vi "FTW-TestStep-Template-Core_Step.vi"(0 "FTW Actor Instance Configuration":string="{\n  \"Identity\": \"ActorName\",\n  \"InboxAddress\": \"inproc://*\",\n  \"LoggerAddress\": \"\",\n  \"My Data\": false,\n  \"Publisher URI\": \"inproc://*\",\n  \"Subscriber URIs\": \"\",\n  \"Refresh Period\": 2\n}", 11 "ErrorIn":errorcluster) -> (15 "Error":errorcluster)   [LabVIEW 2018, in "FTW-TestStep-Template-Core.lvclass"]
uses:
  FTW-TestStep-Template-Core.lvclass
  FTW-TestStep-Template-Core.lvclass/FTW-TestStep-Template-Core.ctl
  source/actor/Instance/FTW-ActorInstance.lvclass/FTW-ActorInstance.ctl
  5377bbb3-02f5-4951-b373-df4eba9c7bf2.vi
  5377bbb3-02f5-4951-b373-df4eba9c7bf2.vi/26df914e-262b-454c-b8ca-6c85922b0070.vi
  C:/Jobs/Featherweight/featherweight-2018/source/actor/Instance/FTW-ActorInstance.lvclass
  source/container/FTW-Container-FromVariant.vi
  source/container/FTW-Container-New-FromContainer.vi
  source/JSON/FTW-JSON-SerializeAndDestroy.vi
  source/actor/JobSequencer/FTW-SEQ-Current.vi
  source/actor/Message/Base/FTW-Message.lvclass
  source/actor/Connector/FTW-ActorConnector.lvclass
  source/actor/Instance/FTW-ActorInstance.lvclass
  source/actor/Message/Request/FTW-Message-IncomingRequest.lvclass
  source/actor/Publisher/FTW-Publisher.lvclass
  source/actor/Subscriber/FTW-Subscriber.lvclass
panel:
  # "#TODO\nhide controls for a GUI"
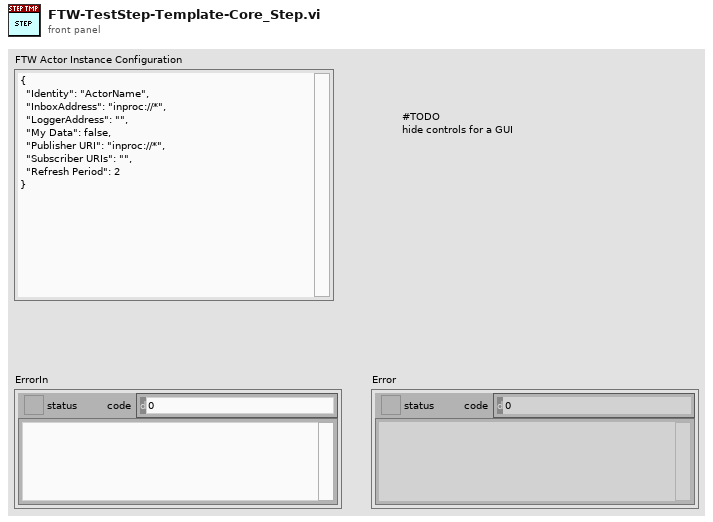
[diagram p1: front panel]
types:
  T1 = cluster{"Incoming Requests":refnum<event-registration>, "Local Messages":refnum<event-registration>, "Subscriber Registration":refnum<event-registration>}
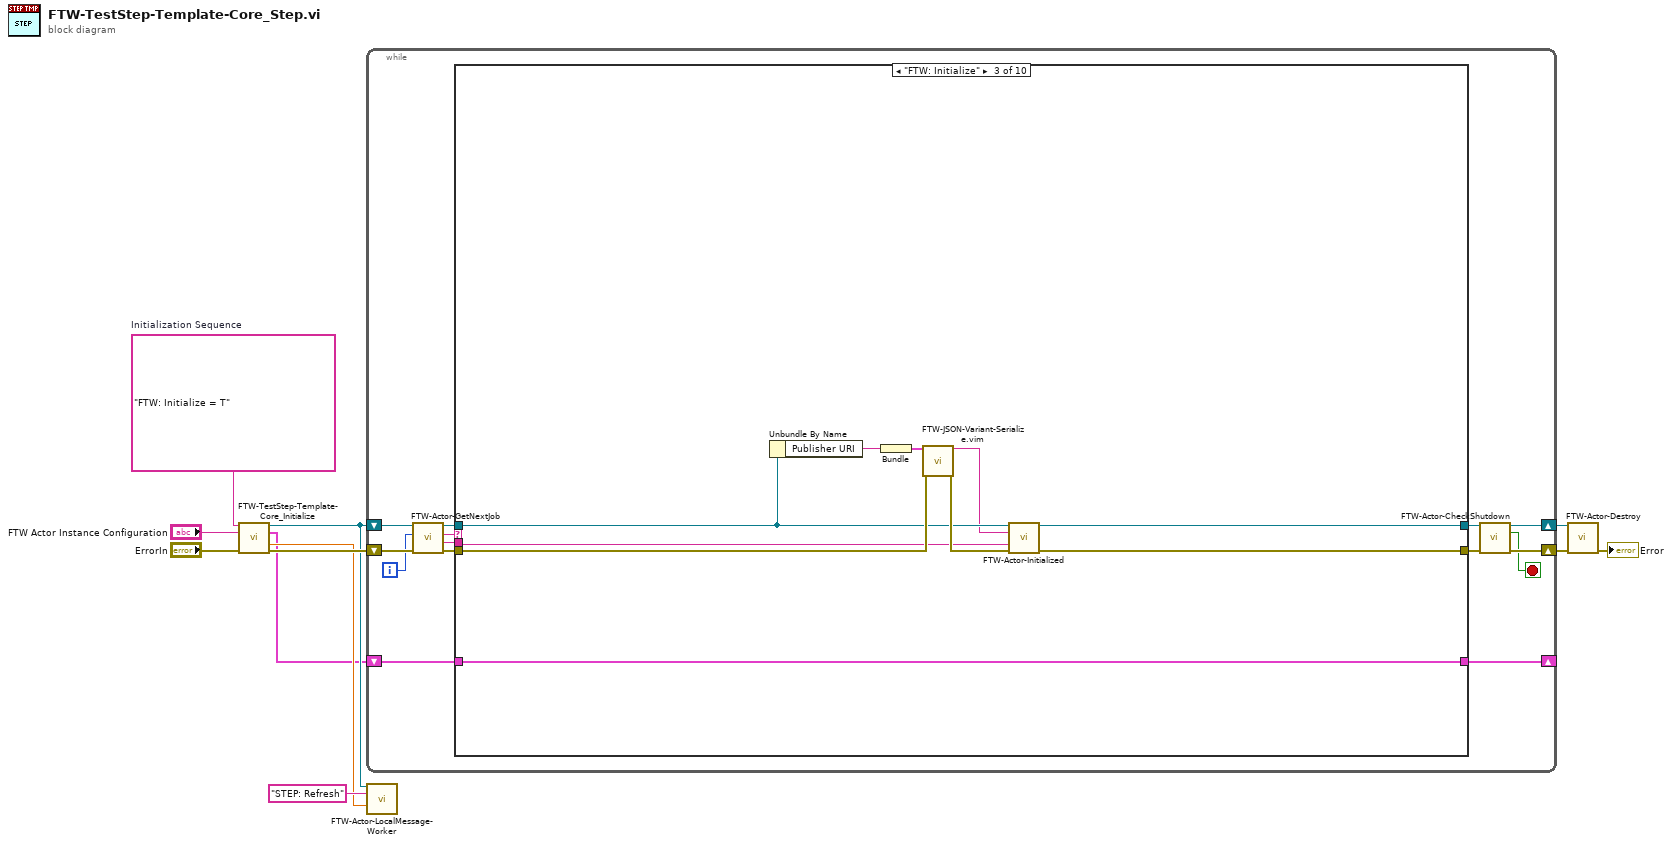
[diagram p0: block diagram]
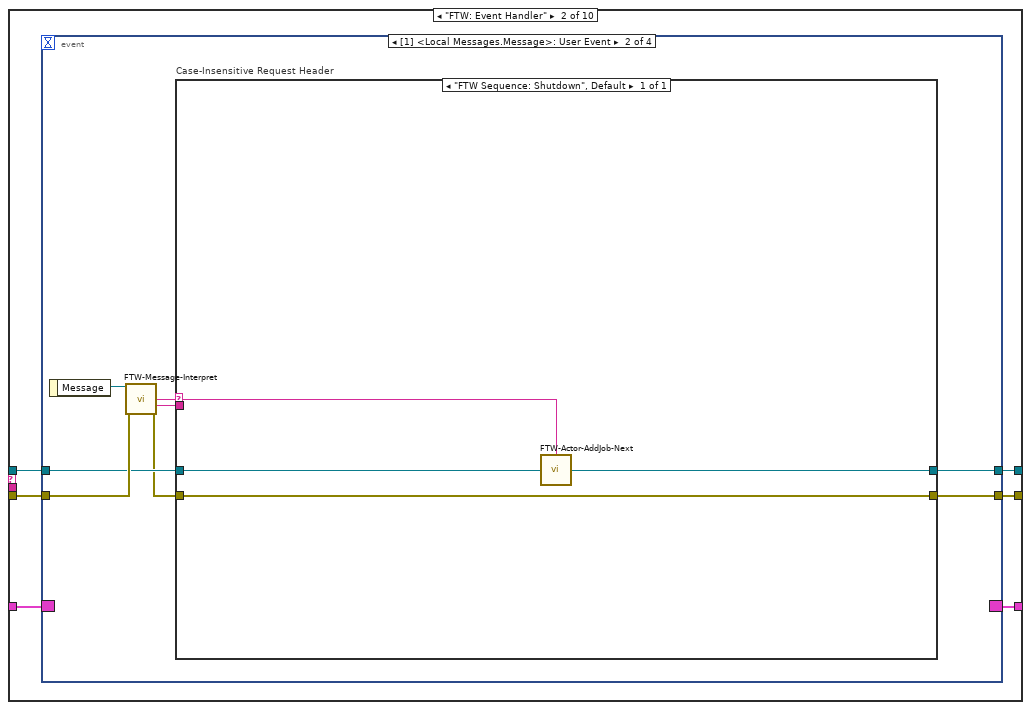
[diagram p3: hidden frame]
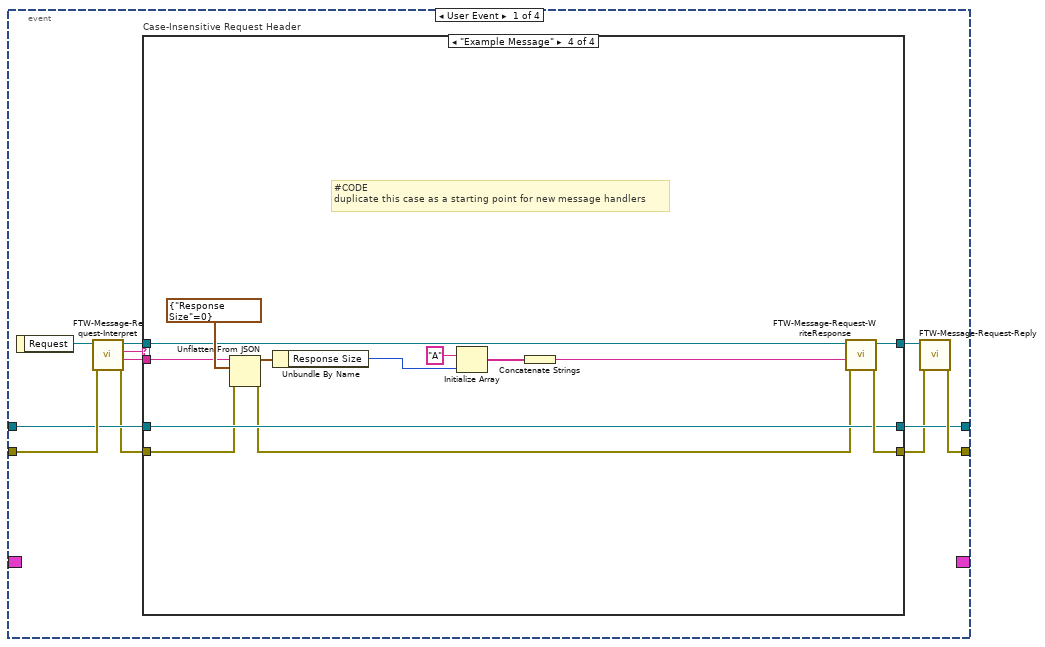
[diagram p4: hidden frame]
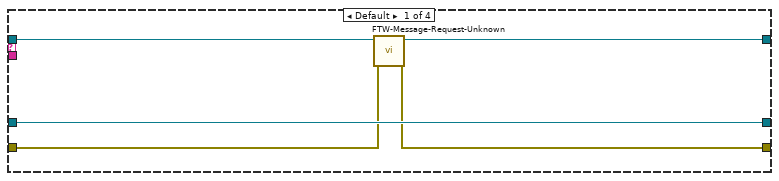
[diagram p5: hidden frame]
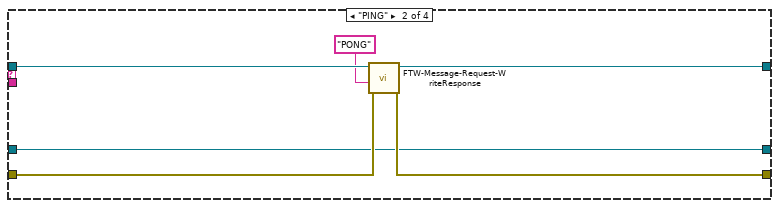
[diagram p6: hidden frame]
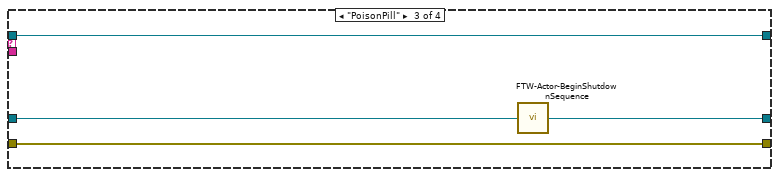
[diagram p7: hidden frame]
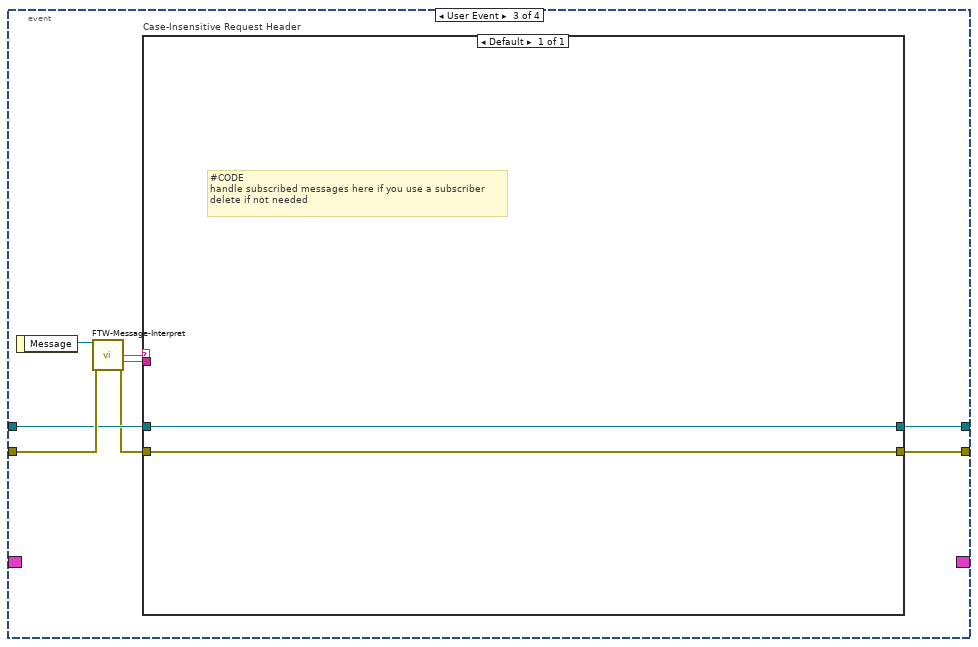
[diagram p8: hidden frame]
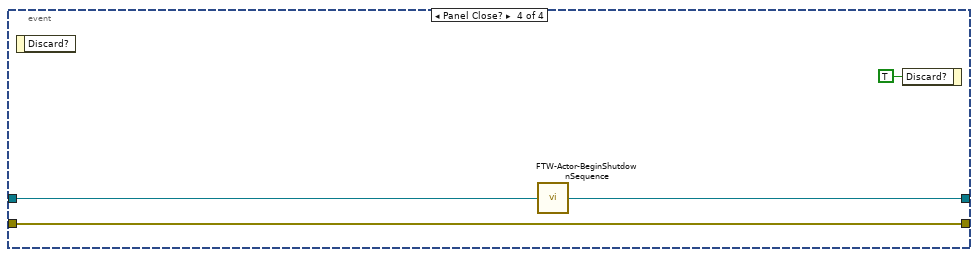
[diagram p9: hidden frame]
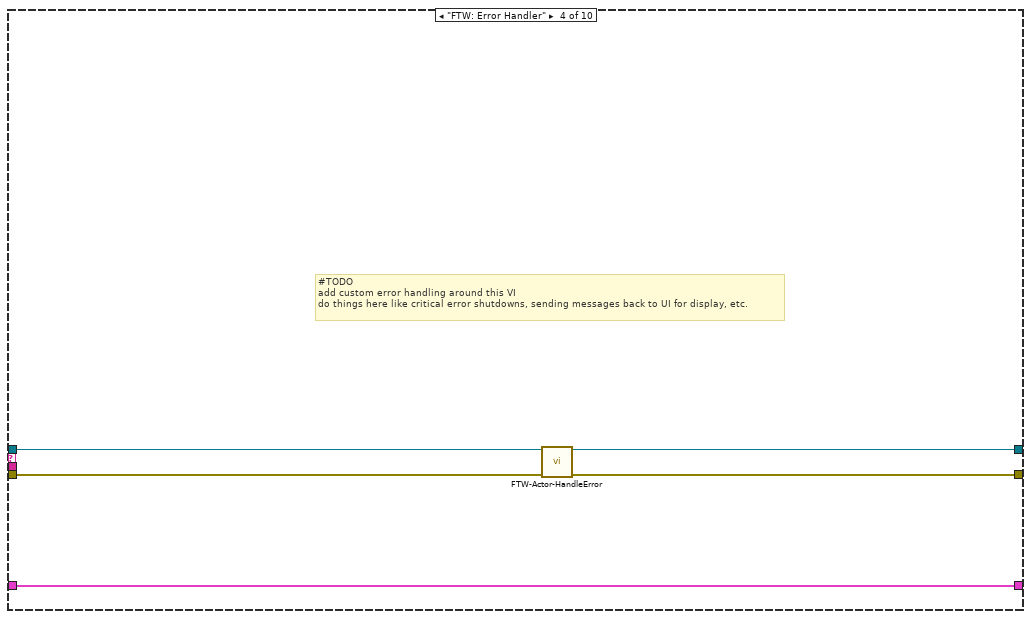
[diagram p10: hidden frame]
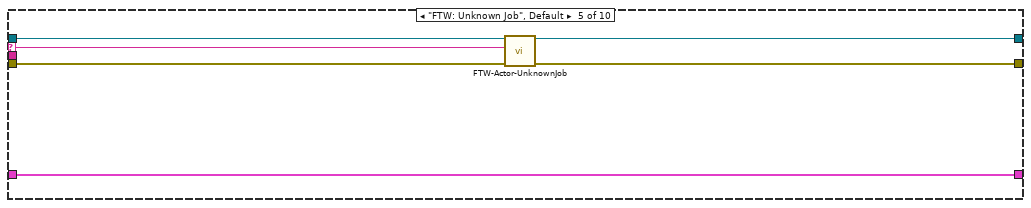
[diagram p11: hidden frame]
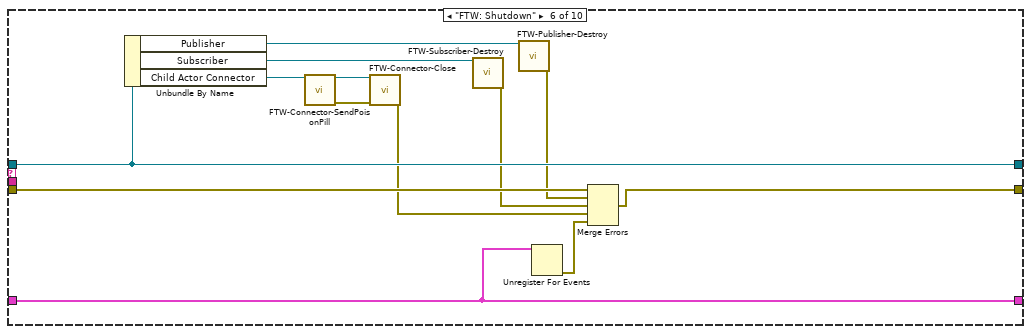
[diagram p12: hidden frame]
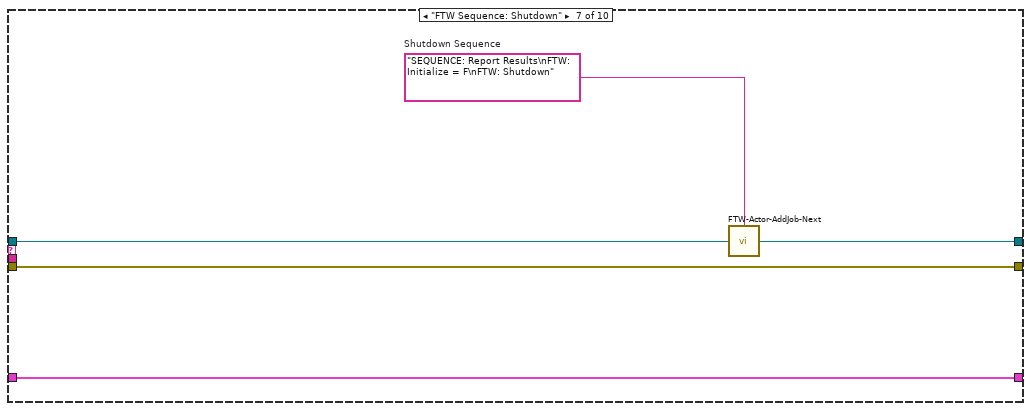
[diagram p13: hidden frame]
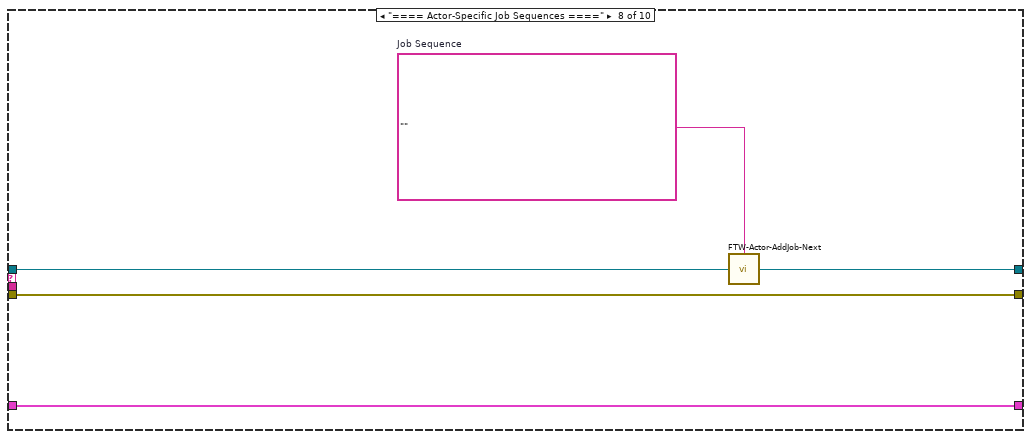
[diagram p14: hidden frame]
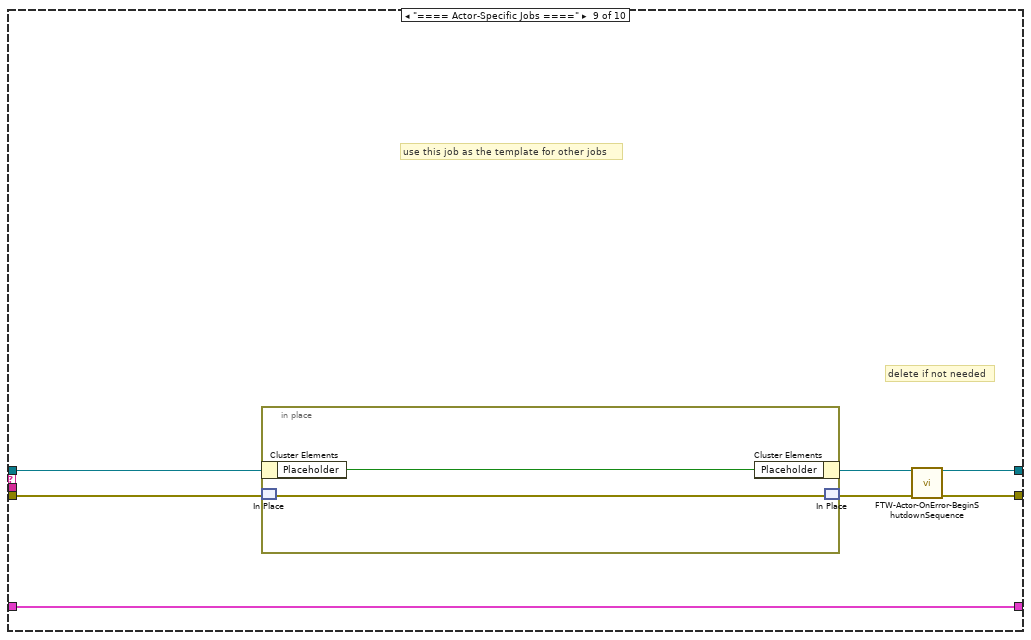
[diagram p15: hidden frame]
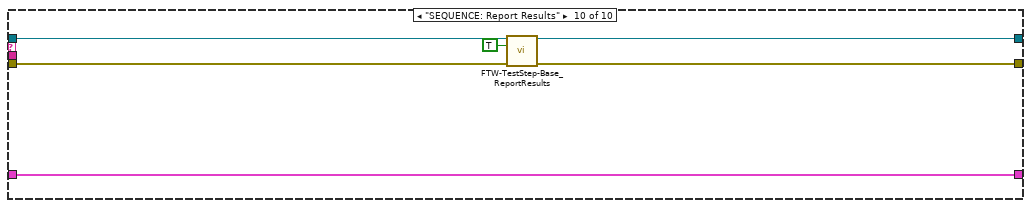
[diagram p16: hidden frame]
diagram:
  w7 = "FTW: Initialize = T"  # Initialization Sequence
  n1 = call "FTW-TestStep-Template-Core_Initialize.vi"("Initialization Sequence"=w7, "FTW Actor Instance Configuration"="FTW Actor Instance Configuration", "error in (no error)"="ErrorIn") -> ("FTW-TestStep-Template-Core Out"=w3:refnum<class "FTW-TestStep-Template-Core.lvclass">, "Event Refnums"=w1:T1, "Refresh Period"=w2:dbl, "error out"=w8:errorcluster)  [unwired: 9 in]
  n2 = while {
    shift-right: [w15] -> w10
    shift-left: w8 -> [w22]
    shift-right: [w12] -> _
    shift-left: w1 -> [w25]
    shift-right: [w17] -> w11
    shift-left: w3 -> [w24]
    i -> [w13]
    stop <- w14 stop-if-true
    n3 = call "FTW-Actor-GetNextJob.vi"("error in"=w22, "Jobs Performed"=w13, "FTW Actor Instance"=w24) -> ("error out"=w21:errorcluster, "Job Data"=w19:string, "Job Name"=w20:string, "FTW Actor Instance out"=w23:refnum<class "FTW-TestStep-Template-Core.lvclass">)  [unwired: 5 in]
    n4 = case shown="\"FTW: Initialize\"" w20 {
      selector: w20 -> [_ _ _ _ w115 _ _ _ _ _]
      tunnel: [w27 w34 w105 w110 w118 w132 w137 w142 w146 w154] -> w16
      tunnel: w21 -> [w27 w33 w109 w112 w119 w133 w137 w142 w149 w157]
      tunnel: w25 -> [w28 w29 w107 w114 w120 w130 w138 w143 w150 w158]
      tunnel: [w28 w32 w107 w114 w120 w130 w138 w143 w150 w158] -> w12
      tunnel: w19 -> [_ _ w102 _ _ _ _ _ _ _]
      tunnel: [w26 w31 w106 w111 w116 w129 w135 w140 w144 w155] -> w18
      tunnel: w23 -> [w26 w30 w104 w113 w117 w129 w136 w141 w147 w156]
      frame "==== Featherweight Framework Jobs ====" {
      }
      frame "FTW: Event Handler" {
        n5 = event shown="[1] <Local Messages.Message>: User Event" {
          selector: w29 -> [_ _ _ _]
          dyn-events: [_ _ _ _] -> w32
          timeout: _ -> [_ _ _ _]
          tunnel: [w44 w76 w88 w98] -> w34
          tunnel: w33 -> [w43 w80 w92 w98]
          tunnel: [w38 w77 w89 w96] -> w31
          tunnel: w30 -> [w42 w79 w91 w97]
          event User Event {
            n6 = event-data() -> ("Request"=w45:refnum<class "FTW-Message-IncomingRequest.lvclass">)  [unwired: 1 in]
            n7 = call "FTW-Message-Request-Interpret.vi"("error in"=w43, "FTW Incoming Request"=w45) -> ("error out"=w41:errorcluster, "Request Body"=w35:string, "Request Header"=w39:string, "FTW Incoming Request out"=w40:refnum<class "FTW-Message-IncomingRequest.lvclass">)  [unwired: 6 in]
            n8 = case "Case-Insensitive Request Header" shown="\"Example Message\"" w39 {
              tunnel: [w48 w54 w59 w73] -> w37
              tunnel: w41 -> [w49 w55 w59 w62]
              tunnel: [w50 w53 w60 w71] -> w38
              tunnel: w42 -> [w50 w53 w58 w71]
              tunnel: w40 -> [w47 w56 w57 w63]
              tunnel: [w46 w52 w57 w72] -> w36
              tunnel: w35 -> [_ _ _ w61]
              frame Default {
                n9 = call "FTW-Message-Request-Unknown.vi"("error in"=w49, "FTW Incoming Request"=w47) -> ("error out"=w48:errorcluster, "FTW Incoming Request Out"=w46:refnum<class "FTW-Message-IncomingRequest.lvclass">)  [unwired: 8 in]
              }
              frame "PING" {
                n10 = call "FTW-Message-Request-WriteResponse.vi"("error in"=w55, "Response Body"="PONG" ("Response Header"), "FTW Incoming Request"=w56) -> ("error out"=w54:errorcluster, "FTW Incoming Request out"=w52:refnum<class "FTW-Message-IncomingRequest.lvclass">)  [unwired: 7 in]
              }
              frame "PoisonPill" {
                n11 = call "FTW-Actor-BeginShutdownSequence.vi"("FTW Actor Instance"=w58) -> ("FTW Actor Instance out"=w60:refnum<class "FTW-TestStep-Template-Core.lvclass">)  [unwired: 3 in]
              }
              frame "Example Message" {
                # "#CODE\nduplicate this case as a starting point for new message handlers"
                n12 = Unflatten From JSON(JSON string=w61, type and defaults=cluster{"Response Size":i32} {"Response Size"=0}, error in (no error)=w62) -> (value=w68:cluster{"Response Size":i32}, error out=w70:errorcluster)  [unwired: 4 in]
                n13 = Unbundle By Name(w68) -> ("Response Size"=w67:i32)
                n14 = Initialize Array("A", w67) -> (w65:string[])
                n15 = Concatenate Strings(w65) -> (w64:string)
                n16 = call "FTW-Message-Request-WriteResponse.vi"("error in"=w70, "Response Body"=w64, "FTW Incoming Request"=w63) -> ("error out"=w73:errorcluster, "FTW Incoming Request out"=w72:refnum<class "FTW-Message-IncomingRequest.lvclass">)  [unwired: 7 in]
              }
            }
            n17 = call "FTW-Message-Request-Reply.vi"("FTW: Reply Error"=w37, "FTW Incoming Request"=w36) -> ("error out"=w44:errorcluster)  [unwired: 8 in, 1 out]
          }
          event User Event {
            n18 = event-data() -> ("Message"=w81:refnum<class "FTW-Message.lvclass">)  [unwired: 1 in]
            n19 = call-dynamic "FTW-Message-Interpret.vi"("FTW Message"=w81, "error in"=w80) -> ("Message Header"=w75:string, "Message Body"=w74:string, "error out"=w78:errorcluster)  [unwired: 9 in, 2 out]
            n20 = case "Case-Insensitive Request Header" shown="\"FTW Sequence: Shutdown\", Default" w75 {
              selector: w75 -> [w82]
              tunnel: [w84] -> w76
              tunnel: w78 -> [w84]
              tunnel: [w83] -> w77
              tunnel: w79 -> [w85]
              tunnel: w74 -> [_]
              frame "FTW Sequence: Shutdown", Default {
                n21 = call "FTW-Actor-AddJob-Next.vi"("Add Next in Job Queue"=w82, "FTW Actor Instance"=w85) -> ("FTW Actor Instance out"=w83:refnum<class "FTW-TestStep-Template-Core.lvclass">)  [unwired: 2 in]
              }
            }
          }
          event User Event {
            n22 = event-data() -> ("Message"=w93:refnum<class "FTW-Message.lvclass">)  [unwired: 1 in]
            n23 = call-dynamic "FTW-Message-Interpret.vi"("FTW Message"=w93, "error in"=w92) -> ("Message Header"=w87:string, "Message Body"=w86:string, "error out"=w90:errorcluster)  [unwired: 9 in, 2 out]
            n24 = case "Case-Insensitive Request Header" shown="Default" w87 {
              tunnel: [w94] -> w88
              tunnel: w90 -> [w94]
              tunnel: [w95] -> w89
              tunnel: w91 -> [w95]
              tunnel: w86 -> [_]
              frame Default {
                # "#CODE\nhandle subscribed messages here if you use a subscriber\ndelete if not needed"
              }
            }
          }
          event Panel Close? {
            n25 = event-data() -> ()  [unwired: 1 in, 1 out]
            n26 = call "FTW-Actor-BeginShutdownSequence.vi"("FTW Actor Instance"=w97) -> ("FTW Actor Instance out"=w96:refnum<class "FTW-TestStep-Template-Core.lvclass">)  [unwired: 3 in]
            n27 = event-data("Discard?"=TRUE) -> ()  [unwired: 1 in, 1 out]
          }
        }
      }
      frame "FTW: Initialize" {
        n28 = Unbundle By Name(w104) -> ("Publisher URI"=w103:string)
        n29 = Bundle("Publisher URI"=w103) -> (w101:cluster{"Publisher URI":string})  [unwired: 1 in]
        n30 = call "FTW-JSON-Variant-Serialize.vim"("Variant"=w101, "error in"=w109) -> ("JSON String"=w100:string, "error out"=w108:errorcluster)  [unwired: 12 in]
        n31 = call-dynamic "FTW-Actor-Initialized.vi"("FTW Actor Instance"=w104, "Initialized Response"=w100, "Positive Init?"=w102, "error in"=w108) -> ("FTW Actor Instance out"=w106:refnum<class "FTW-TestStep-Template-Core.lvclass">, "error out"=w105:errorcluster)  [unwired: 10 in]
      }
      frame "FTW: Error Handler" {
        # "#TODO\nadd custom error handling around this VI\ndo things here like critical error shutdowns, sending messages back to UI for display, etc."
        n32 = call-dynamic "FTW-Actor-HandleError.vi"("FTW Actor Instance"=w113, "error in"=w112) -> ("FTW Actor Instance out"=w111:refnum<class "FTW-TestStep-Template-Core.lvclass">, "error out"=w110:errorcluster)  [unwired: 10 in, 2 out]
      }
      frame "FTW: Unknown Job", Default {
        n33 = call-dynamic "FTW-Actor-UnknownJob.vi"("FTW Actor Instance"=w117, "Unknown Job"=w115, "error in"=w119) -> ("FTW Actor Instance out"=w116:refnum<class "FTW-TestStep-Template-Core.lvclass">, "error out"=w118:errorcluster)  [unwired: 11 in]
      }
      frame "FTW: Shutdown" {
        n34 = Unbundle By Name(w129) -> ("Publisher"=w128:refnum<class "FTW-Publisher.lvclass">, "Subscriber"=w126:refnum<class "FTW-Subscriber.lvclass">, "Child Actor Connector"=w124:refnum<class "FTW-ActorConnector.lvclass">)
        n35 = call-dynamic "FTW-Connector-SendPoisonPill.vi"("FTW Actor Connector"=w124) -> ("FTW Actor Connector out"=w123:refnum<class "FTW-ActorConnector.lvclass">, "error out"=w122:errorcluster)  [unwired: 9 in, 4 out]
        n36 = call-dynamic "FTW-Connector-Close.vi"("FTW Actor Connector"=w123, "error in"=w122) -> ("error out"=w121:errorcluster)  [unwired: 13 in]
        n37 = call "FTW-Subscriber-Destroy.vi"("FTW-Subscription In"=w126) -> ("error out"=w125:errorcluster)  [unwired: 14 in]
        n38 = call "FTW-Publisher-Destroy.vi"("FTW-Publisher In"=w128) -> ("error out"=w127:errorcluster)  [unwired: 14 in]
        n39 = Unregister For Events(event registration refnum=w130) -> (error out=w131:errorcluster)  [unwired: 1 in]
        n40 = Merge Errors(w133, w127, w125, w121, w131) -> (w132:errorcluster)
      }
      frame "FTW Sequence: Shutdown" {
        w134 = "SEQUENCE: Report Results\nFTW: Initialize = F\nFTW: Shutdown"  # Shutdown Sequence
        n41 = call "FTW-Actor-AddJob-Next.vi"("Add Next in Job Queue"=w134, "FTW Actor Instance"=w136) -> ("FTW Actor Instance out"=w135:refnum<class "FTW-TestStep-Template-Core.lvclass">)  [unwired: 2 in]
      }
      frame "==== Actor-Specific Job Sequences ====" {
        w139 = ""  # Job Sequence
        n42 = call "FTW-Actor-AddJob-Next.vi"("Add Next in Job Queue"=w139, "FTW Actor Instance"=w141) -> ("FTW Actor Instance out"=w140:refnum<class "FTW-TestStep-Template-Core.lvclass">)  [unwired: 2 in]
      }
      frame "==== Actor-Specific Jobs ====" {
        # "delete if not needed"
        # "use this job as the template for other jobs"
        n43 = in-place {
          n44 = in-place-cluster #1(w147) -> ("Placeholder"=w151:bool)
          n45 = in-place-match #2(w149) -> (w152:errorcluster)
          n46 = in-place-cluster #1("Placeholder"=w151) -> (w145:refnum<class "FTW-TestStep-Template-Core.lvclass">)
          n47 = in-place-match #2(w152) -> (w148:errorcluster)
        }
        n48 = call-dynamic "FTW-Actor-OnError-BeginShutdownSequence.vi"("FTW Actor Instance"=w145, "error in"=w148) -> ("FTW Actor Instance out"=w144:refnum<class "FTW-TestStep-Template-Core.lvclass">, "error out"=w146:errorcluster)  [unwired: 12 in]
      }
      frame "SEQUENCE: Report Results" {
        n49 = call-dynamic "FTW-TestStep-Base_ReportResults.vi"("FTW-TestStep-Base In"=w156, "Passed"=TRUE, "error in (no error)"=w157) -> ("FTW-TestStep-Base Out"=w155:refnum<class "FTW-TestStep-Template-Core.lvclass">, "error out"=w154:errorcluster)  [unwired: 11 in]
      }
    }
    n50 = call "FTW-Actor-CheckShutdown.vi"("FTW Actor Instance"=w18, "error in"=w16) -> ("FTW Actor Instance out"=w17:refnum<class "FTW-TestStep-Template-Core.lvclass">, "Shutdown?"=w14:bool, "error out"=w15:errorcluster)  [unwired: 11 in]
  }
  n51 = call "FTW-Actor-LocalMessage-Worker.vi"("FTW-ActorInstance In"=w3, "Message Header"="STEP: Refresh", "Send Rate"=w2) -> ()  [unwired: 13 in]
  n52 = call-dynamic "FTW-Actor-Destroy.vi"("FTW Actor Instance"=w11, "error in"=w10) -> ("error out"=→"Error":errorcluster)  [unwired: 13 in]
